vi "Validate Sequence.vi"(8 "error in (no error)":refnum<class "MultiErrors.lvclass">, 11 "Sequence Config in":refnum<class "Sequence Config.lvclass">) -> (0 "error out":refnum<class "MultiErrors.lvclass">, 3 "Sequence Config out":refnum<class "Sequence Config.lvclass">)   [LabVIEW 2020, in "VolatusSeq.lvlib" / "Sequence Validation.lvclass"]
uses:
  Sequence Validation.lvclass
  VolatusErrorUtilities/MultiErrors/MultiErrors.lvclass
  Sequence Config/Sequence Config.lvclass
  VolatusErrorUtilities/MultiErrors/MultiErrors.lvclass/MultiErrors.ctl
  Sequence Validation.lvclass/Sequence Validation.ctl
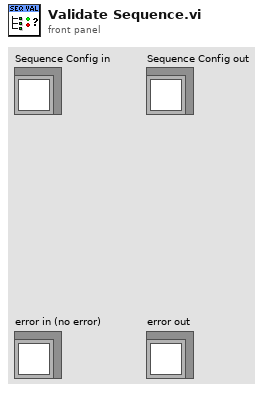
[diagram p1: front panel]
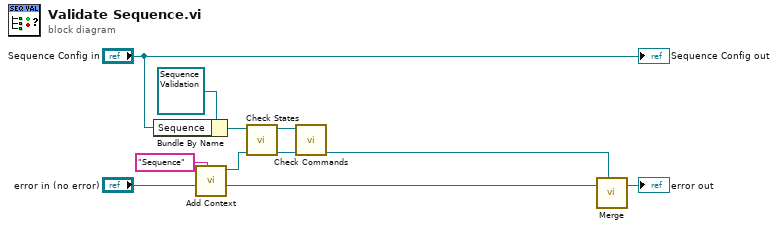
[diagram p0: block diagram]
diagram:
  n1 = Bundle By Name(cluster=refnum<class "Sequence Validation.lvclass"> refnum ("Sequence Validation in"), "Sequence"="Sequence Config in") -> (w7:refnum<class "Sequence Validation.lvclass">)
  n2 = call "Add Context.vi"("Context"="Sequence", "MultiErrors in"="error in (no error)") -> ("Original Context"=w9:refnum<class "MultiErrors.lvclass">, "Added Context"=w6:refnum<class "MultiErrors.lvclass">)  [unwired: 8 in]
  n3 = call "Check States.vi"("error in (no error)"=w6, "Sequence Validation in"=w7) -> ("error out"=w4:refnum<class "MultiErrors.lvclass">, "Sequence Validation out"=w3:refnum<class "Sequence Validation.lvclass">)  [unwired: 8 in]
  n4 = call "Check Commands.vi"("error in (no error)"=w4, "Sequence Validation in"=w3) -> ("error out"=w2:refnum<class "MultiErrors.lvclass">)  [unwired: 8 in, 1 out]
  n5 = call "Merge.vi"("First Error In"=w9, "Second Error In"=w2) -> ("MultiErrors out"=→"error out":refnum<class "MultiErrors.lvclass">)  [unwired: 5 in]
  "Sequence Config out" <- "Sequence Config in"
